vi "Update Template Files.vi"(8 "error in (no error)":errorcluster, 11 "Server Library (Library Item) in":refnum<vi>) -> (0 "error out":errorcluster, 3 "Server Library (Library Item) out":refnum<vi>)   [LabVIEW 2019, in "gRPC Template Creation Utility.lvlib"]
uses:
  gRPC Template Creation Utility.lvlib
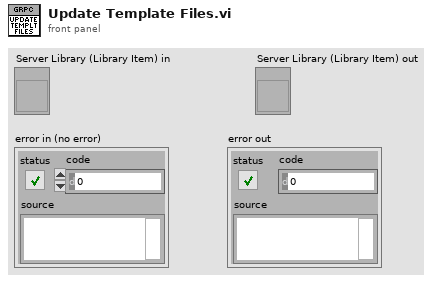
[diagram p1: front panel]
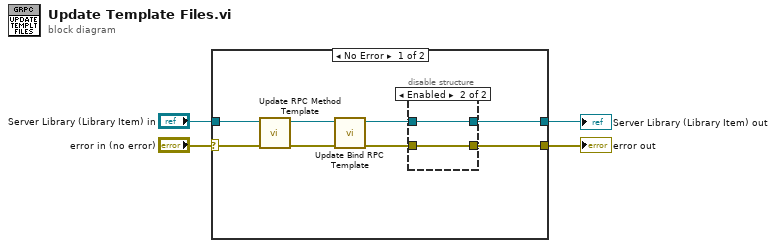
[diagram p0: block diagram]
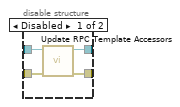
[diagram p2: hidden frame]
diagram:
  n1 = case shown="No Error" "error in (no error)" {
    selector: "error in (no error)" -> [w11 w20]
    tunnel: "Server Library (Library Item) in" -> [w12 w19]
    tunnel: [w6 w20] -> w2
    tunnel: [w5 w19] -> w1
    frame No Error {
      n2 = call "Update RPC Method Template.vi"("error in (no error)"=w11, "Server Library (Library Item) in"=w12) -> ("error out"=w10:errorcluster, "Server Library (Library Item) out"=w9:refnum<vi>)  [unwired: 8 in]
      n3 = call "Update Bind RPC Template.vi"("error in (no error)"=w10, "Server Library (Library Item) in"=w9) -> ("error out"=w8:errorcluster, "Server Library (Library Item) out"=w7:refnum<vi>)  [unwired: 8 in]
      n4 = disable-structure shown="Enabled" {
        disable-tunnel: w8 -> [w16 w17]
        disable-tunnel: w7 -> [w15 w18]
        disable-tunnel: [w14 w17] -> w6
        disable-tunnel: [w13 w18] -> w5
        frame Disabled {
          n5 = call "Update RPC Template Accessors.vi"("error in"=w16, "Server Library (Library Item) in"=w15) -> ("error out"=w14:errorcluster, "Server Library (Library Item) out"=w13:refnum<vi>)  [unwired: 8 in]
        }
        frame Enabled {
        }
      }
    }
    frame Error {
    }
  }
  "Server Library (Library Item) out" <- w1
  "error out" <- w2
